vi "Mischer_pot_preassure_correction.vi"(0 "Pot [mbar]":dbl format="%_3e") -> (1 "Pot corrected [mbar]":dbl format="%#_3g", 2 "TemperaturePot [K]":dbl format="%#_3g")   [LabVIEW 2018]
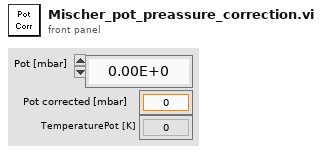
[diagram p1: front panel]
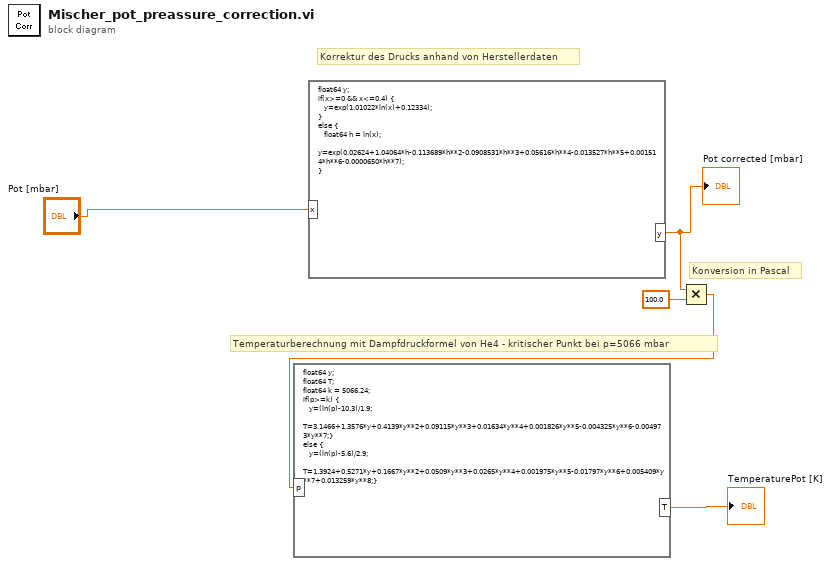
[diagram p0: block diagram]
diagram:
  # "Konversion in Pascal"
  # "Temperaturberechnung mit Dampfdruckformel von He4 - kritischer Punkt bei p=5066 mbar"
  # "Korrektur des Drucks anhand von Herstellerdaten"
  n1 = formula code="float64 y;\nif(x>=0 && x<=0.4) {\n   y=exp(1.01022*ln(x)+0.12334);\n}\nelse {\n   float64 h = ln(x);\n   y=exp(0.02624+1.04064*h-0.113689*h**2-0.0908531*h**3+0.05616*h**4-0.013527*h**5+0.001514*h**6-0.0000650*h**7);\n}"("x"="Pot [mbar]") -> ("y"=w4:dbl)
  "Pot corrected [mbar]" <- w4
  n2 = Multiply(x=w4, y=100.0) -> (x*y=w3:dbl)
  n3 = formula code="float64 y;\nfloat64 T;\nfloat64 k = 5066.24;\nif(p>=k) {\n   y=(ln(p)-10.3)/1.9;\n   T=3.1466+1.3576*y+0.4139*y**2+0.09115*y**3+0.01634*y**4+0.001826*y**5-0.004325*y**6-0.004973*y**7;}\nelse {\n   y=(ln(p)-5.6)/2.9;\n   T=1.3924+0.5271*y+0.1667*y**2+0.0509*y**3+0.0265*y**4+0.001975*y**5-0.01797*y**6+0.005409*y**7+0.013259*y**8;}"("p"=w3) -> ("T"=→"TemperaturePot [K]":dbl)
